vi "进账管理.vi"() -> ()   [LabVIEW 2010]
panel:
  in  "查询":bool
  in  "结束时间":timestamp
  in  "起始时间":timestamp
  in  "按时间查询":bool
  in  "返回":bool
  in  "确定按钮":bool
  in  "进账明细":string
  in  "进账金额":dbl
  in  "进账人":string
  in  "进账时间":timestamp
  in  "进账记录":string[][](table)
  # "进账管理界面"
  # "进账查询"
  # "进账操作"
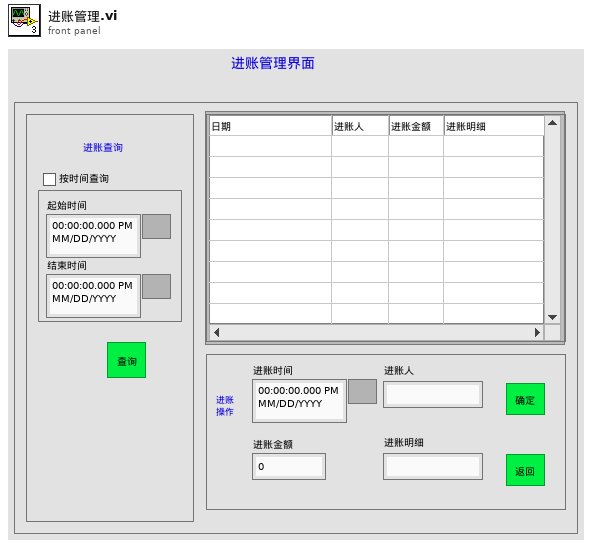
[diagram p1: front panel]
types:
  T1 = cluster{u64, "进账人":string, "进账金额":dbl, "进账明细":string}
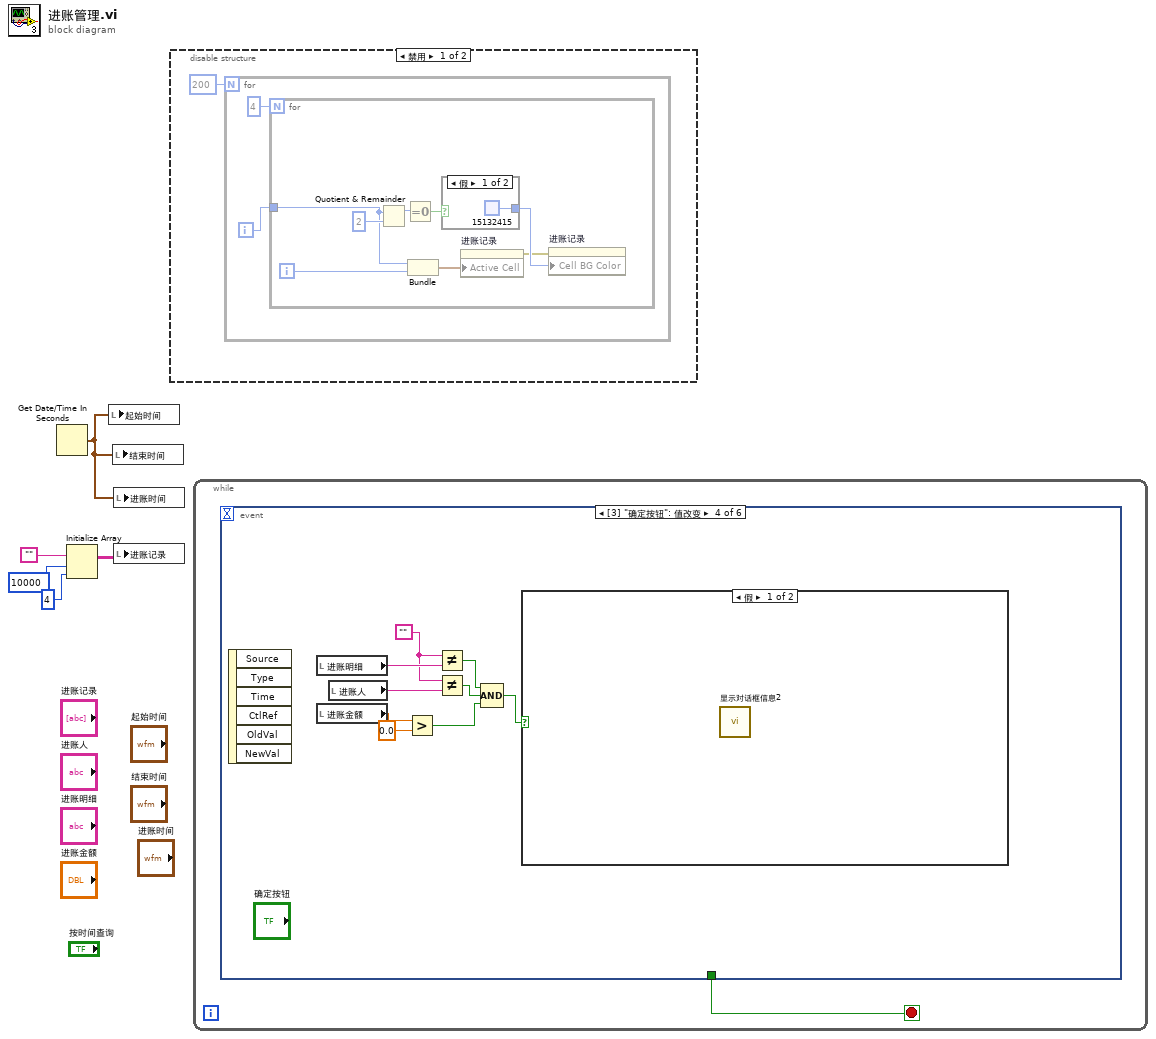
[diagram p0: block diagram]
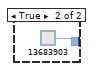
[diagram p2: hidden frame]
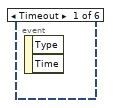
[diagram p4: hidden frame]
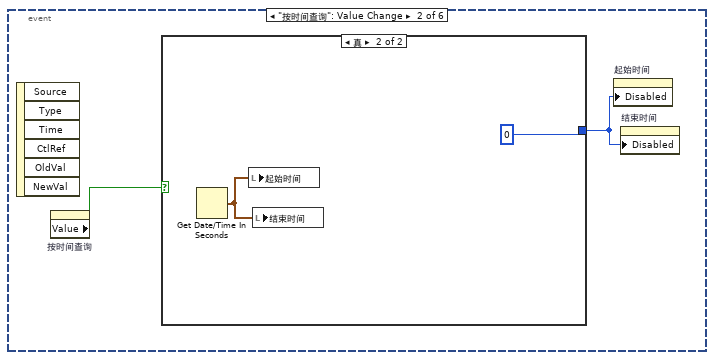
[diagram p5: hidden frame]
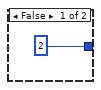
[diagram p6: hidden frame]
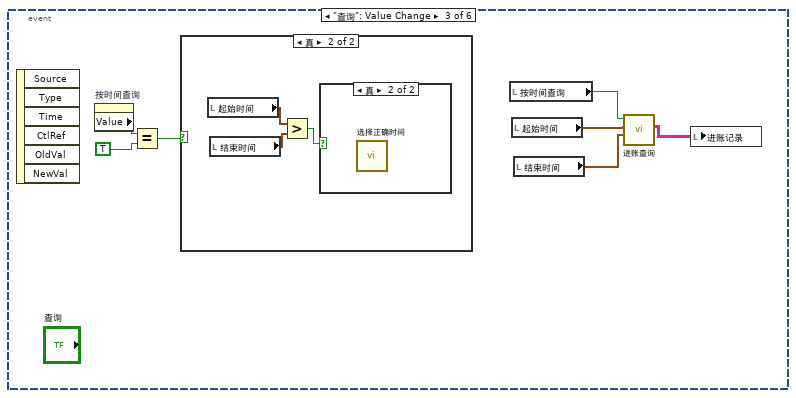
[diagram p7: hidden frame]
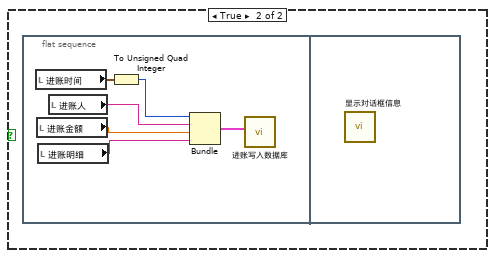
[diagram p10: hidden frame]
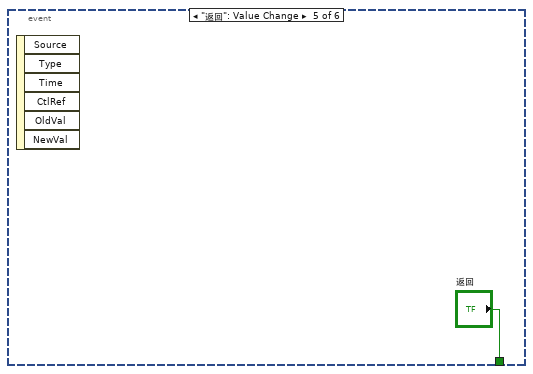
[diagram p11: hidden frame]
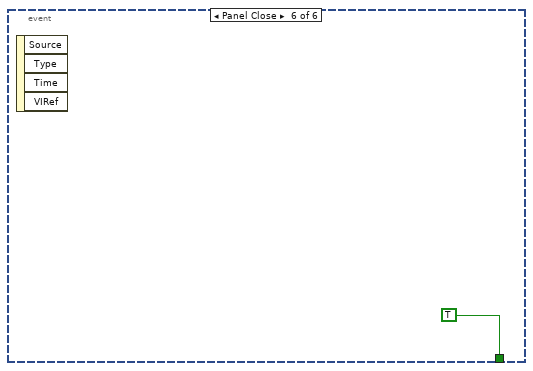
[diagram p12: hidden frame]
diagram:
  n1 = Get Date/Time In Seconds() -> (seconds since 1Jan1904=w5:timestamp)
  n2 = Initialize Array("", 10000, 4 ("维数大小")) -> (w4:string[][])
  n3 = local write "起始时间"(w5) -> ()
  n4 = local write "结束时间"(w5) -> ()
  n5 = local write "进账时间"(w5) -> ()
  n6 = local write "进账记录"(w4) -> ()
  n7 = disable-structure shown="禁用" {
    frame Disabled {
      n8 = for {
        N: 200 -> [_]
        i -> [w7]
        n9 = for {
          N: 4 -> [_]
          tunnel: w7 -> [w9]
          i -> [w10]
          n10 = Quotient & Remainder(x=w9, y=2) -> (x-y*floor(x/y)=w12:i32)  [unwired: 1 out]
          n11 = Equal To 0?(x=w12) -> (x = 0?=w13:bool)
          n12 = Bundle(w9, w10) -> (w14:cluster{i32, i32})  [unwired: 1 in]
          n13 = case shown="假" w13 {
            tunnel: [u32 15132415 u32 13683903] -> w16
            frame False {
            }
            frame True {
            }
          }
          n14 = property on="进账记录" class="Tbl (严格)"("Active Cell"=w14) -> (error out=w11:errorcluster)  [unwired: 2 in, 1 out]
          n15 = property on="进账记录" class="Tbl (严格)"(error in=w11, "Cell BG Color"=w16) -> ()  [unwired: 1 in, 2 out]
        }
      }
    }
    frame Enabled {
    }
  }
  n16 = while {
    stop <- w19 stop-if-true
    n17 = event shown="[3] \"确定按钮\": 值改变" {
      selector: _ -> [_ _ _ _ _ _]
      dyn-events: _ -> [_ _ _ _ _ _]
      timeout: _ -> [_ _ _ _ _ _]
      tunnel: [_ _ _ _ "返回" TRUE] -> w19
      event Timeout {
        n18 = event-data() -> ()  [unwired: 1 in, 2 out]
      }
      event "按时间查询": Value Change {
        n19 = event-data() -> ()  [unwired: 1 in, 6 out]
        n20 = property on="按时间查询" class="Bool (严格)"() -> ("Value"=w20:bool)  [unwired: 2 in, 2 out]
        n21 = case shown="真" w20 {
          tunnel: [2 0] -> w21
          frame False {
          }
          frame True {
            n22 = Get Date/Time In Seconds() -> (seconds since 1Jan1904=w24:timestamp)
            n23 = local write "起始时间"(w24) -> ()
            n24 = local write "结束时间"(w24) -> ()
          }
        }
        n25 = property on="起始时间" class="AbsTime (严格)"("Disabled"=w21) -> ()  [unwired: 2 in, 2 out]
        n26 = property on="结束时间" class="AbsTime (严格)"("Disabled"=w21) -> ()  [unwired: 2 in, 2 out]
      }
      event "查询": Value Change {
        n27 = event-data() -> ()  [unwired: 1 in, 6 out]
        n28 = property on="按时间查询" class="Bool (严格)"() -> ("Value"=w30:bool)  [unwired: 2 in, 2 out]
        n29 = Equal?(x=w30, y=TRUE) -> (x = y?=w29:bool)
        n30 = case shown="真" w29 {
          frame False {
          }
          frame True {
            n31 = local read "起始时间"() -> (w33:timestamp)
            n32 = local read "结束时间"() -> (w32:timestamp)
            n33 = Greater?(x=w33, y=w32) -> (0:w34:bool)
            n34 = case shown="真" w34 {
              frame False {
              }
              frame True {
                n35 = call "选择正确时间"() -> ()  [unwired: 10 in, 2 out]
              }
            }
          }
        }
        n36 = local read "按时间查询"() -> (w27:bool)
        n37 = local read "起始时间"() -> (w26:timestamp)
        n38 = local read "结束时间"() -> (w25:timestamp)
        n39 = call "进账查询.vi"("结束时间"=w25, "起始时间"=w26, "可选条件"=w27) -> ("查询结果"=w28:string[][])  [unwired: 8 in]
        n40 = local write "进账记录"(w28) -> ()
      }
      event "确定按钮": Value Change {
        w42 = ""
        n41 = event-data() -> ()  [unwired: 1 in, 6 out]
        n42 = local read "进账明细"() -> (w43:string)
        n43 = local read "进账金额"() -> (w40:dbl)
        n44 = local read "进账人"() -> (w41:string)
        n45 = Greater?(x=w40, y=0.0) -> (0:w36:bool)
        n46 = Not Equal?(x=w42, y=w43) -> (x != y?=w38:bool)
        n47 = Not Equal?(x=w42, y=w41) -> (x != y?=w37:bool)
        n48 = Compound Arithmetic op=AND(w38, w37, w36) -> (w35:bool)
        n49 = case shown="假" w35 {
          frame False {
            n50 = call "显示对话框信息2"() -> ()  [unwired: 10 in, 2 out]
          }
          frame True {
            n51 = flat-sequence {
              frame #0 {
                n52 = local read "进账时间"() -> (w49:timestamp)
                n53 = local read "进账金额"() -> (w46:dbl)
                n54 = local read "进账明细"() -> (w45:string)
                n55 = local read "进账人"() -> (w47:string)
                n56 = To Unsigned Quad Integer(1:w49) -> (0:w48:u64)
                n57 = Bundle(w48, "进账人"=w47, "进账金额"=w46, "进账明细"=w45) -> (w44:T1)  [unwired: 1 in]
                n58 = call "进账写入数据库.vi"("输出簇"=w44) -> ()  [unwired: 11 in]
              }
              frame #1 {
                n59 = call "显示对话框信息"() -> ()  [unwired: 10 in, 2 out]
              }
            }
          }
        }
      }
      event "返回": Value Change {
        n60 = event-data() -> ()  [unwired: 1 in, 6 out]
      }
      event Panel Close {
        n61 = event-data() -> ()  [unwired: 1 in, 4 out]
      }
    }
  }
